vi "Write fifo config.vi"(8 "error in (no error)":errorcluster, 10 "fifo config":T1, 11 "fifo channel in":refnum<class "fifo channel.lvclass">) -> (0 "error out":errorcluster, 3 "fifo channel out":refnum<class "fifo channel.lvclass">)   [LabVIEW 2014, in "fifo channel.lvclass"]
uses:
  fifo channel.lvclass
  fifo channel settings.ctl
  fifo channel.lvclass/fifo channel.ctl
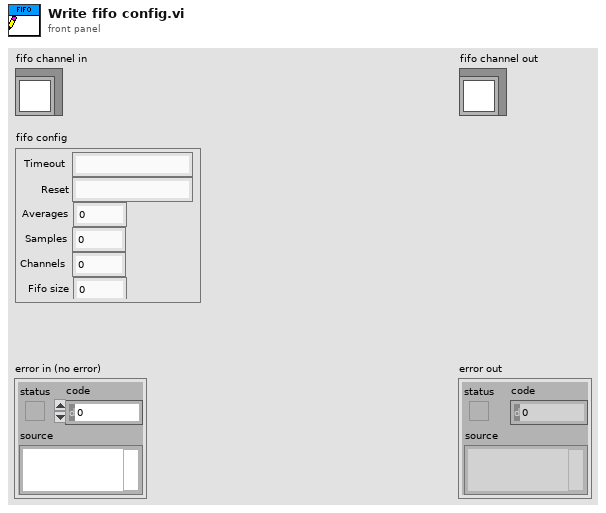
[diagram p1: front panel]
types:
  T1 = typedef "fifo channel.lvclass/fifo channel settings.ctl" = cluster{"Timeout":string, "Reset":string, "Averages":i32, "Samples":u32, "Channels":i32, "Fifo size":u32}
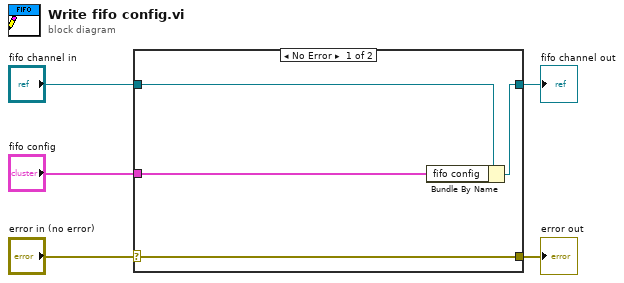
[diagram p0: block diagram]
diagram:
  n1 = case shown="No Error" "error in (no error)" {
    selector: "error in (no error)" -> [w9 w10]
    tunnel: [w9 w10] -> w4
    tunnel: [w7 w11] -> w2
    tunnel: "fifo channel in" -> [w8 w11]
    tunnel: "fifo config" -> [w6 _]
    frame No Error {
      n2 = Bundle By Name(cluster=w8, "fifo config"=w6) -> (w7:refnum<class "fifo channel.lvclass">)
    }
    frame Error {
    }
  }
  "error out" <- w4
  "fifo channel out" <- w2
